vi "Set AWG Volts.vi"(0 "Semiconductor Module Context":T1, 5 "error in (no error)":errorcluster, 6 "Pins":string[](array[string]), 9 "Script":string="script myScript\n  generate myWaveform\nend script") -> (14 "Semiconductor Module Context Out":T1, 19 "error out":errorcluster)   [LabVIEW 2013]
uses:
  <vilib>/NI_TestStand_SemiconductorModule/NI_TestStand_Semiconductor_Module.lvlibp/PinMap/General/SemiconductorModuleContext.ctl
  <vilib>/NI_TestStand_SemiconductorModule/NI_TestStand_Semiconductor_Module.lvlibp
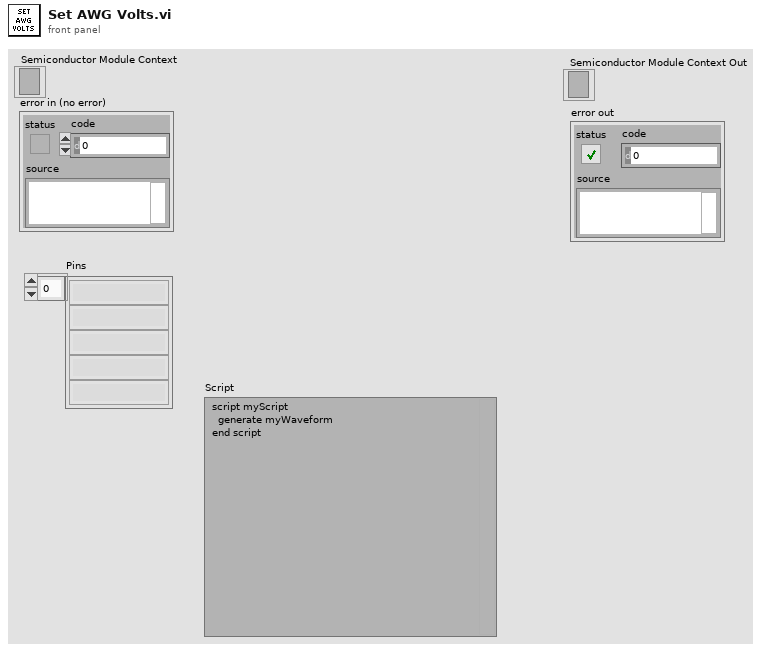
[diagram p1: front panel]
types:
  T1 = typedef "NI_TestStand_Semiconductor_Module.lvlibp/SemiconductorModuleContext.ctl" = refnum<k7>
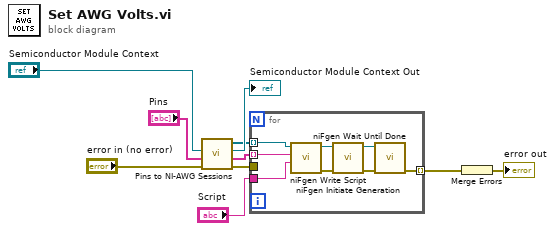
[diagram p0: block diagram]
diagram:
  n1 = call "Pins to NI-AWG Sessions.vi"("error in (no error)"="error in (no error)", "Pins"="Pins", "Semiconductor Module Context"="Semiconductor Module Context") -> ("error out"=w4:errorcluster, "Channel Lists"=w6:string[], "Semiconductor Module Context Out"=→"Semiconductor Module Context Out":T1, "Instrument Sessions"=w5:refnum<k15>[])  [unwired: 5 in]
  n2 = for {
    tunnel: w6 -> [w14] mode=indexing
    tunnel: w5 -> [w15] mode=indexing
    tunnel: w4 -> [_]
    tunnel: [w12] -> w3 mode=indexing
    tunnel: "Script" -> [w16]
    n3 = call <instrlib>:"niFgen Write Script.vi"("Script"=w16, "Channel Name"=w14, "Instrument Handle"=w15) -> ("error out"=w17:errorcluster, "Instrument Handle Out"=w18:refnum<k15>)  [unwired: 7 in]
    n4 = call <instrlib>:"niFgen Initiate Generation.vi"("error in (no error)"=w17, "Instrument Handle"=w18) -> ("error out"=w13:errorcluster, "Instrument Handle Out"=w11:refnum<k15>)  [unwired: 8 in]
    n5 = call <instrlib>:"niFgen Wait Until Done.vi"("error in (no error)"=w13, "Instrument Handle"=w11) -> ("error out"=w12:errorcluster)  [unwired: 8 in, 1 out]
  }
  n6 = Merge Errors(w3) -> (→"error out":errorcluster)
